vi "Read Init VI.vi"(8 "Error In":errorcluster caption="error in", 11 "Custom Device .NET Ref In":refnum<k24>) -> (0 "Error Out":errorcluster caption="error in", 2 "Initialization VI Properties":T1, 3 "Custom Device .NET Ref Out":refnum<k24>)   [LabVIEW 2019, in "VeriStand Custom Device XML Parser.lvlib"]
doc: "Reads and returns the properties of the custom device initialization VI"
uses:
  VeriStand Custom Device XML Parser.lvlib
  NationalInstruments.VeriStand.XMLReader
  XML Controls/Initialization VI Properties.ctl
  XML Controls/Execution Types.ctl
  XML Controls/Path Cluster.ctl
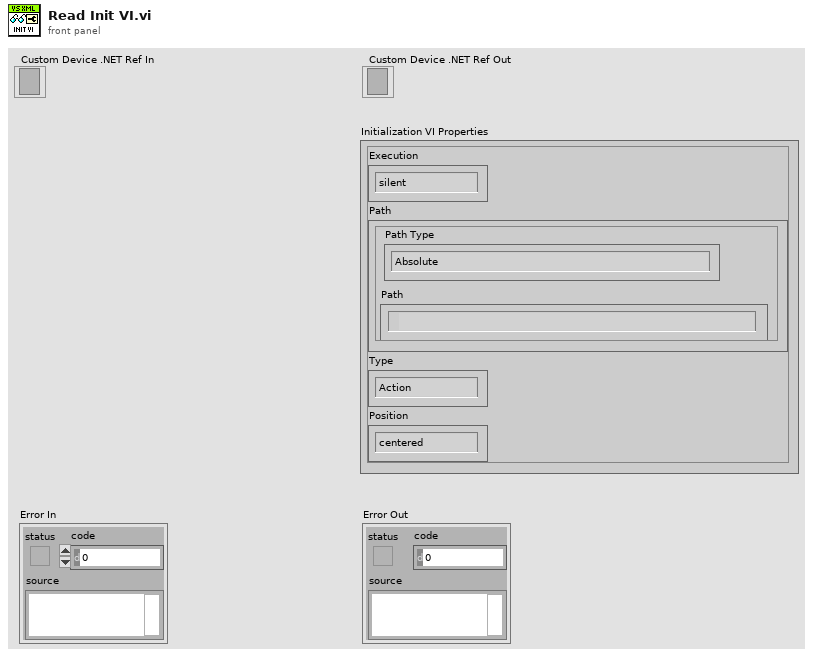
[diagram p1: front panel]
types:
  T1 = typedef "VeriStand Custom Device XML Parser.lvlib/Initialization VI Properties.ctl" = cluster{"Execution":T2, "Path":T3, "Type":enum16{"Action", "VI"}, "Position":enum16{"centered", "mouse pointer"}}
  T2 = typedef "VeriStand Custom Device XML Parser.lvlib/Execution Types.ctl" = enum16{"silent", "modal", "floating", "default"}
  T3 = typedef "VeriStand Custom Device XML Parser.lvlib/Path Cluster.ctl" = cluster{"Path":path, "Path Type":enum16{"Absolute", "To Base", "To Common Doc Dir", "To Application Data Dir"}}
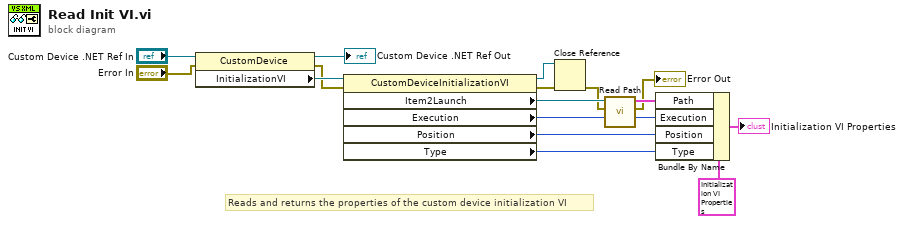
[diagram p0: block diagram]
diagram:
  # "Reads and returns the properties of the custom device initialization VI"
  n1 = property class="CustomDevice"(reference="Custom Device .NET Ref In", error in="Error In") -> (reference out=→"Custom Device .NET Ref Out":refnum<k24>, error out=w13:errorcluster, "InitializationVI"=w14:refnum<k24>)
  n2 = property class="CustomDeviceInitializationVI"(reference=w14, error in=w13) -> (reference out=w11:refnum<k24>, error out=w10:errorcluster, "Item2Launch"=w9:refnum<k24>, "Execution"=w8:i32, "Position"=w7:i32, "Type"=w6:i32)
  n3 = Close Reference(reference=w11, error in (no error)=w10) -> (error out=w1:errorcluster)
  n4 = call "Read Path.vi"("Error In"=w1, "Path .NET Ref"=w9) -> ("Error Out"=→"Error Out":errorcluster, "Path Properties"=w3:T3)  [unwired: 8 in]
  n5 = Bundle By Name(cluster=T1 {"Execution"=enum."silent", "Path"={"Path"=path "", "Path Type"=enum."Absolute"}, "Type"=enum."Action", "Position"=enum."centered"} ("Initialization VI Properties"), "Path"=w3, "Execution"=w8, "Position"=w7, "Type"=w6) -> (→"Initialization VI Properties":T1)
